vi "DAQmx task create-Encoder trigger.vi"(10 "Internal O/P reference of the \ncounter used as the AO clock":tag, 11 "Data length":i32) -> (0 "error out":errorcluster, 1 "Encoder trigger DO sequence":digitaldata, 2 "# points in output waveform":i32, 3 "Refnum out":refnum<k21>)   [LabVIEW 2013]
uses:
  <vilib>/DAQmx/write.llb/DAQmx Write (Digital Wfm 1Chan NSamp).vi
  <vilib>/DAQmx/create/channels.llb/DAQmx Create Channel (DO-Digital Output).vi
  Global Variables/General Globals.vi
  <vilib>/DAQmx/configure/timing.llb/DAQmx Timing (Sample Clock).vi
  <vilib>/Waveform/DWDTOps.llb/DWDT Uncompress Digital.vi
  <vilib>/DAQmx/miscellaneous.llb/DAQmx Fill In Error Info.vi
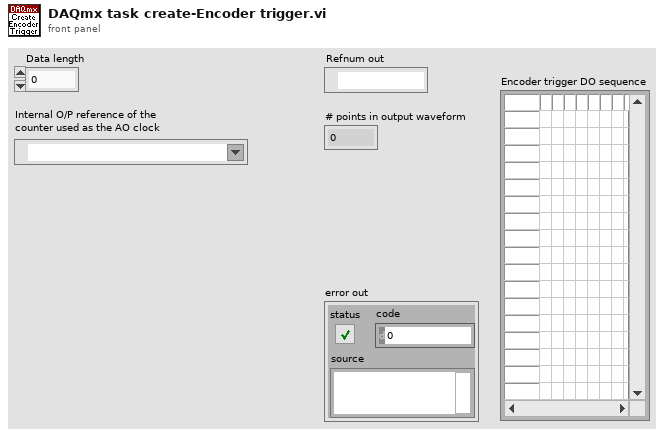
[diagram p1: front panel]
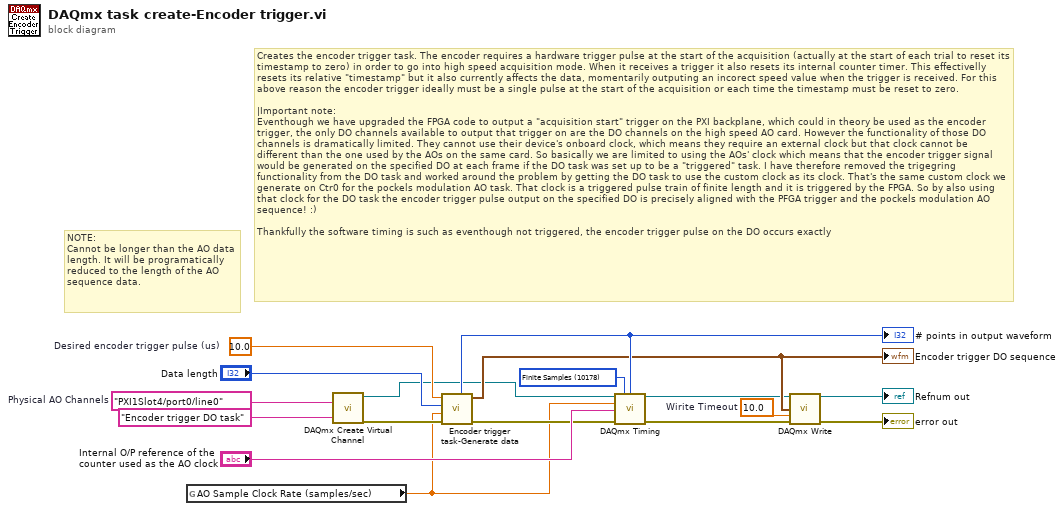
[diagram p0: block diagram]
diagram:
  w6 = 10178 items=["Finite Samples"=10178, "Continuous Samples"=10123] ("sample mode")
  w7 = 10.0  # Wirite Timeout
  w14 = 10.0  # Desired encoder trigger pulse (us)
  w12 = tag "PXI1Slot4/port0/line0"  # Physical AO Channels
  # "Creates the encoder trigger task. The encoder requires a hardware trigger pulse at the start of the acquisition (actually at the start of each trial to reset its timestamp to zero) in order to go into high speed acquisition mode. When it receives a trigger it also resets its internal counter timer. This effectivelly resets its relative \"timestamp\" but it also currently affects the data, momentarily outputing an incorect speed value when the trigger is received. For this above reason the encoder trigger ideally must be a single pulse at the start of the acquisition or each time the timestamp must be reset to zero.\n\n|Important note: \nEventhough we have upgraded the FPGA code to output a \"acquisition start\" trigger on the PXI backplane, which could in theory be used as the encoder trigger, the only DO channels available to output that trigger on are the DO channels on the high speed AO card. However the functionality of those DO channels is dramatically limited. They cannot use their device's onboard clock, which means they require an external clock but that clock cannot be different than the one used by the AOs on the same card. So basically we are limited to using the AOs' clock which means that the encoder trigger signal would be generated on the specified DO at each frame if the DO task was set up to be a \"triggered\" task. I have therefore removed the trigegring functionality from the DO task and worked around the problem by getting the DO task to use the custom clock as its clock. That's the same custom clock we generate on Ctr0 for the pockels modulation AO task. That clock is a triggered pulse train of finite length and it is triggered by the FPGA. So by also using that clock for the DO task the encoder trigger pulse output on the specified DO is precisely aligned with the PFGA trigger and the pockels modulation AO sequence! :)\n\nThankfully the software timing is such as eventhough not triggered, the encoder trigger pulse on the DO occurs exactly"
  # "NOTE:\nCannot be longer than the AO data length. It will be programatically reduced to the length of the AO sequence data."
  n1 = global read "General Globals.vi" "AO Sample Clock Rate (samples/sec)"() -> (w1:dbl)
  n2 = call-poly <vilib>:"DAQmx Create Virtual Channel.vi"("lines"=w12, "name to assign"="Encoder trigger DO task") -> ("task out"=w5:refnum<k21>, "error out"=w8:errorcluster)  [unwired: 12 in]
  n3 = call "Encoder trigger task-Generate data.vi"("error in (no error)"=w8, "Sample Clock Rate"=w1, "Number of samples in pockels modulation AO sequence"="Data length", "Specified encoder trigger pulse width (us)"=w14) -> ("error"=w4:errorcluster, "Encoder trigger DO sequence"=w10:digitaldata, "# points in output waveform"=w17:i32)  [unwired: 1 in, 4 out]
  "# points in output waveform" <- w17
  "Encoder trigger DO sequence" <- w10
  n4 = call-poly <vilib>:"DAQmx Timing.vi"("task/channels in"=w5, "sample mode"=w6, "samples per channel"=w17, "rate"=w1, "source"="Internal O/P reference of the \ncounter used as the AO clock", "error in"=w4) -> ("task out"=w3:refnum<k21>, "error out"=w2:errorcluster)  [unwired: 8 in]
  n5 = call-poly <vilib>:"DAQmx Write.vi"("task/channels in"=w3, "data"=w10, "timeout"=w7, "error in"=w2) -> ("task out"=→"Refnum out":refnum<k21>, "error out"=→"error out":errorcluster)  [unwired: 9 in, 1 out]
